vi "MAIN_change_valve_position.vi"(8 "error in":errorcluster, 9 "variant":variant, 10 "Start acquisition":bool, 11 "queue valve":refnum<queue>) -> (0 "error out":errorcluster, 1 "Valve ready?":bool, 3 "Next task":T1, 4 "Valve H":u8(knob)=1 min=1 max=22 scale=1.0..22.0, 5 "Valve position OUT":u8)   [LabVIEW 2015]
uses:
  CONTROLS/Q_main_element.ctl
  CONTROLS/Q_VALVE_element.ctl
  GLOBAL/Global_VALVE.vi
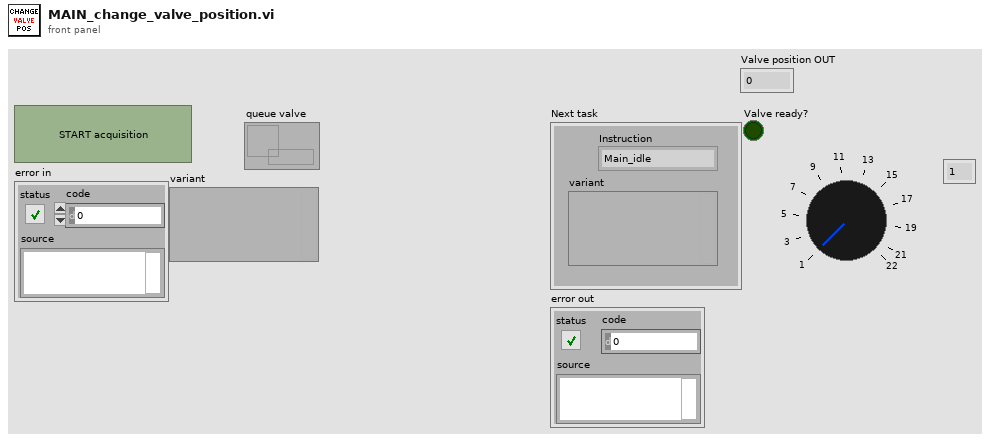
[diagram p1: front panel]
types:
  T1 = typedef "Q_main_element.ctl" = cluster{"variant":variant, "Instruction":enum16{"Main_idle", "Main_initialize", "Main_initialize_TDMS", "Main_initialize_Queue", "Main_error", "Main_DAQ_initialization_results", "Main_ASI_initialization_results", "Main_Piezo_initialization_results", "Main_Valve_initialization_results", "Main_Pump_initialization_results", "Main_CAMERA_initialization_results", "Main_FPGA_initialization_results", "Main_DAQ_error", "Main_ASI_error", "Main_Piezo_error", "Main_CAMERA_error", "Main_Valve_error", "Main_Pump_error", "Main_FPGA_error", "Main_start_acquiring", "Main_not_acquiring", "Main_acquiring", "Main_stop_acquiring", "Main_change_exposure", "Main_change_z_scan_parameters", "Main_define_ROI", "Main_define_mosaic", "Main_read_kinetic_time", "Main_cooler", "Main_read_temperature", "Main_save_XY", "Main_load_XY", "Main_discard_XY", "Main_move_to_XY", "Main_measure_QPD", "Main_autofocus_calibration", "Main_autofocus_initialization", "Main_autofocus_stop", "Main_save_PID", "Main_change_H_valve_position", "Main_two_way_valve", "Main_save_movie", "Main_init_single_scan", "Main_single_scan", "Main_stop_single_scan", "Main_merFISH_illumination_parameters", "Main_merFISH_buffer_probe_list", "Main_merFISH_injections_procedure", "Main_merFISH_save_setpoint", "Main_merFISH_DAPI_parameters", "Main_merFISH_Brightfield_parameters", "Main_merFISH_save_embryo_ROI", "Main_merFISH_init", "Main_merFISH_resume", "Main_merFISH_start_autofocus", "Main_merFISH_open_close_valve_merFISH", "Main_merFISH_open_close_valve_photobleaching", "Main_merFISH_hybridization", "Main_merFISH_move_to_ROI", "Main_merFISH_wait_stabilization", "Main_merFISH_move_to_REF", "Main_merFISH_scan", "Main_merFISH_photobleaching_injection", "Main_merFISH_photobleaching", "Main_merFISH_send_email", "Main_merFISH_close", "Main_STOP"}}
  T2 = typedef "Q_VALVE_element.ctl" = cluster{"variant":variant, "Instruction":enum16{"VALVE_idle", "VALVE_initialize", "VALVE_error", "VALVE_security_stop", "VALVE_change_position", "VALVE_two_way_valves", "VALVE_init_merFISH", "VALVE_stop"}}
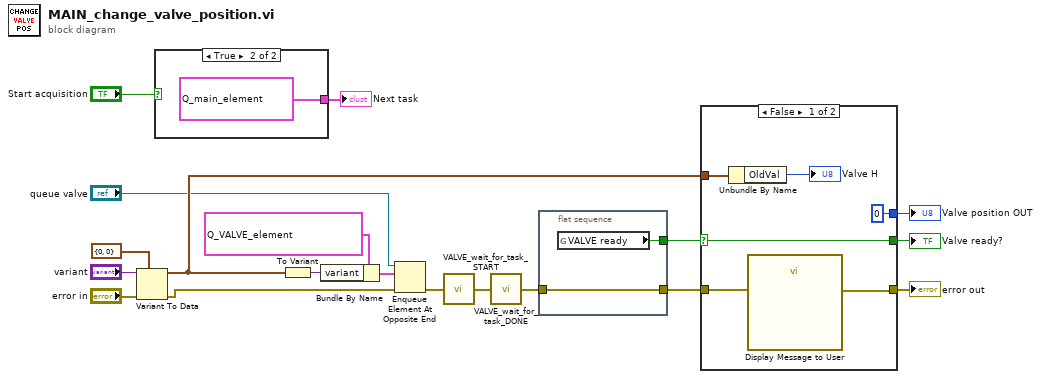
[diagram p0: block diagram]
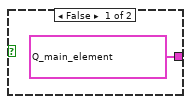
[diagram p2: hidden frame]
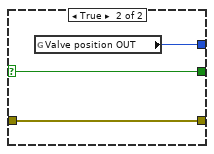
[diagram p3: hidden frame]
diagram:
  n1 = Variant To Data(error in="error in", type=cluster{"Valve H":u8, "OldVal":u8} {"Valve H"=0, "OldVal"=0} ("output cluster"), Variant="variant") -> (data=w18:cluster{"Valve H":u8, "OldVal":u8}, error out=w9:errorcluster)
  n2 = case shown="True" "Start acquisition" {
    tunnel: [T1 {"variant"=variant, "Instruction"=enum."Main_not_acquiring"} ("Q_main_element") T1 {"variant"=variant, "Instruction"=enum."Main_acquiring"} ("Q_main_element")] -> w5
    frame False {
    }
    frame True {
    }
  }
  "Next task" <- w5
  n3 = To Variant(anything=w18) -> (Variant=w11:variant)
  n4 = Bundle By Name(cluster=T2 {"variant"=variant, "Instruction"=enum."VALVE_change_position"} ("element"), "variant"=w11) -> (w12:T2)
  n5 = Enqueue Element At Opposite End(queue="queue valve", element=w12, error in (no error)=w9) -> (error out=w13:errorcluster)  [unwired: 1 in, 2 out]
  n6 = call "VALVE_wait_for_task_START.vi"("error in"=w13) -> ("error out"=w14:errorcluster)
  n7 = call "VALVE_wait_for_task_DONE.vi"("error in"=w14) -> ("error out"=w15:errorcluster)
  n8 = flat-sequence {
    tunnel: w15 -> [w23]
    tunnel: [w23] -> w17
    tunnel: [w22] -> w16
    frame #0 {
      n9 = global read "Global_VALVE.vi" "VALVE ready"() -> (w22:bool)
    }
  }
  n10 = case shown="False" w16 {
    selector: w16 -> [w24 w30]
    tunnel: w17 -> [w29 w32]
    tunnel: [w28 w32] -> w3
    tunnel: w18 -> [w27 _]
    tunnel: [u8 0 ("Valve position OUT") w31] -> w19
    tunnel: [w24 w30] -> w2
    frame False {
      n11 = Unbundle By Name(w27) -> ("OldVal"=→"Valve H":u8)
      n12 = call "Display Message to User"("error in (no error)"=w29) -> ("error out"=w28:errorcluster)  [unwired: 9 in, 1 out]
    }
    frame True {
      n13 = global read "Global_VALVE.vi" "Valve position OUT"() -> (w31:u8)
    }
  }
  "Valve position OUT" <- w19
  "error out" <- w3
  "Valve ready?" <- w2
